vi "Write Ramp Current.vi"(8 "error in":errorcluster, 10 "Current_Ramp":dbl, 11 "57XX in":refnum<class "57XX.lvclass">) -> (0 "error out":errorcluster, 3 "57XX out":refnum<class "57XX.lvclass">)   [LabVIEW 2019, in "57XX.lvlib" / "57XX.lvclass"]
uses:
  Library/57XX.lvclass
  C:/Users/Public/Documents/Development/builds/Engine/Monitored Actor.lvlibp/Monitored Actor/Monitored Actor/Monitored Actor.lvclass
  builds/Engine/Monitored Actor.lvlibp/Monitored Actor/Monitored Actor/Read Actor Label.vi
  builds/Instruments/PowerSupply.lvlibp/Library/PowerSupply.lvclass
  <vilib>/ErrorRing/Error Ring.xnode
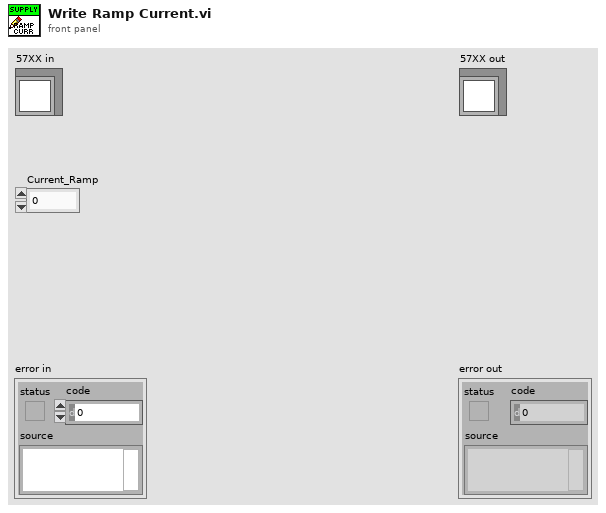
[diagram p1: front panel]
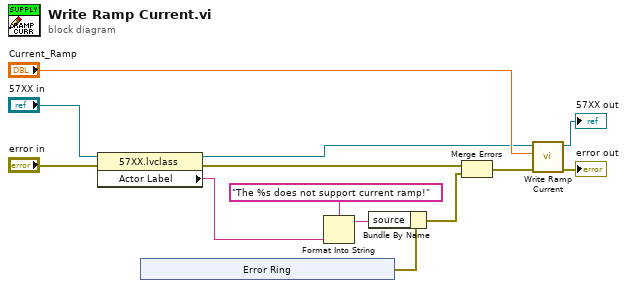
[diagram p0: block diagram]
diagram:
  n1 = property class="57XX.lvclass"(reference="57XX in", error in="error in") -> (reference out=w3:refnum<class "57XX.lvclass">, error out=w10:errorcluster, "Actor Label"=w6:string)
  n2 = xnode "Error Ring"() -> ("error out"=w9:errorcluster)
  n3 = Format Into String(format string="The %s does not support current ramp!", w6) -> (resulting string=w8:string)  [unwired: 2 in, 1 out]
  n4 = Bundle By Name(cluster=w9, "source"=w8) -> (w7:errorcluster)
  n5 = Merge Errors(w10, w7) -> (w1:errorcluster)
  n6 = call-parent "Write Ramp Current.vi"("error in"=w1, "Current_Ramp"="Current_Ramp", "PowerSupply in"=w3) -> ("error out"=→"error out":errorcluster, "PowerSupply out"=→"57XX out":refnum<class "57XX.lvclass">)  [unwired: 7 in]
